vi "Liquid Crystal Display.vi"(0 "LINX Resource In":T1, 1 "string":string, 2 "Clear LCD?":u16, 3 "Data":u8[](array[numeric]), 4 "string 2":string, 5 "Error In":errorcluster) -> (14 "LINX Resource Out":T1, 15 "string":string, 17 "Response":u8[](array[numeric]), 18 "string 2":string, 19 "Error Out":errorcluster)   [LabVIEW 2020]
doc: "Creates a text to be displayed to LCD using the Arduino IDE."
uses:
  <vilib>/MakerHub/LINX/Private/Type Defs/LINX Ref.ctl
  <vilib>/MakerHub/LINX/Private/Type Defs/Platform.ctl
  <vilib>/MakerHub/LINX/Private/Type Defs/Interface.ctl
  <vilib>/MakerHub/LINX/Private/Device/Type Defs/LINX Device Config.ctl
  <vilib>/MakerHub/LINX/Private/Device/Type Defs/TCP Config.ctl
  <vilib>/MakerHub/LINX/Private/Device/Type Defs/Channels.ctl
  <vilib>/MakerHub/LINX/LMH-LINX.lvlib
  <vilib>/MakerHub/LINX/Private/Device/Device.lvlib
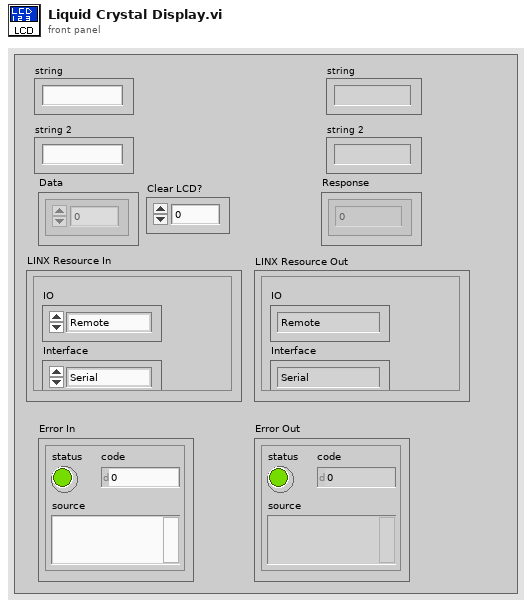
[diagram p1: front panel]
types:
  T1 = typedef "LMH-LINX.lvlib/LINX Ref.ctl" = cluster{"IO":T2, "Interface":T3, "LINX Device Config":T4}
  T2 = typedef "LMH-LINX.lvlib/Platform.ctl" = enum16{"Remote", "Local"}
  T3 = typedef "LMH-LINX.lvlib/Interface.ctl" = enum16{"Serial", "TCP"}
  T4 = typedef "LMH-LINX.lvlib/Device.lvlib/LINX Device Config.ctl" = cluster{"Interface":T3, "COM Port":refnum<visa-resource-name>, "TCP Configuration":T5, "Device Family":u8, "Device ID":u8, "Device Name":string, "TCP Ref":refnum<k5>, "Channels":T6}
  T5 = typedef "LMH-LINX.lvlib/Device.lvlib/TCP Config.ctl" = cluster{"IP Address":string, "Port":u16}
  T6 = typedef "LMH-LINX.lvlib/Channels.ctl" = cluster{"DI":u8[], "DO":u8[], "AI":u8[], "AO":u8[], "PWM":u8[], "QE":u8[], "UART":u8[], "I2C 2":u8[], "SPI":u8[], "CAN":u8[], "Servo":u8[], "AI Ref (V)":dbl, "AI Resolution (Bits)":u8, "AO Ref (V)":dbl, "AO Resolution (Bits)":u8}
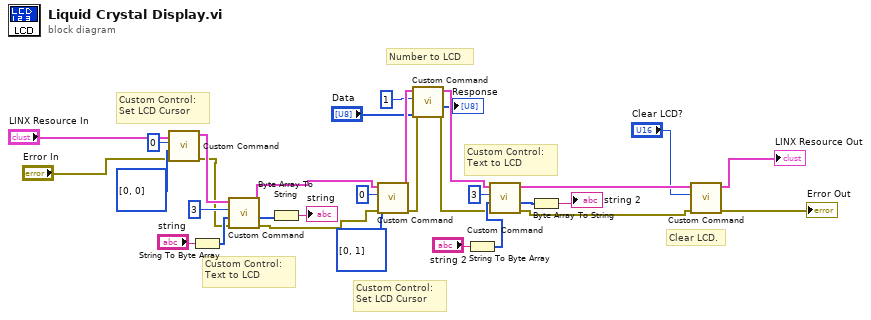
[diagram p0: block diagram]
diagram:
  # "Clear LCD."
  # "Number to LCD"
  # "Custom Control:\nText to LCD"
  # "Custom Control:\nSet LCD Cursor"
  # "Custom Control:\nText to LCD"
  # "Custom Control:\nSet LCD Cursor"
  n1 = call <vilib>:"Custom Command.vi"("Error In"="Error In", "Data"=u8[] [0, 0], "Custom Command Number"=u16 0, "LINX Resource"="LINX Resource In") -> ("Error Out"=w26:errorcluster, "LINX Resource"=w30:T1)  [unwired: 4 in, 2 out]
  n2 = String To Byte Array(string="string") -> (unsigned byte array=w27:u8[])
  n3 = call <vilib>:"Custom Command.vi"("Error In"=w26, "Data"=w27, "Custom Command Number"=u16 3, "LINX Resource"=w30) -> ("Error Out"=w16:errorcluster, "Response"=w25:u8[], "LINX Resource"=w15:T1)  [unwired: 4 in, 1 out]
  n4 = Byte Array To String(unsigned byte array=w25) -> (string=→"string":string)
  n5 = call <vilib>:"Custom Command.vi"("Error In"=w16, "Data"=u8[] [0, 1], "Custom Command Number"=u16 0, "LINX Resource"=w15) -> ("Error Out"=w9:errorcluster, "LINX Resource"=w12:T1)  [unwired: 4 in, 2 out]
  n6 = call <vilib>:"Custom Command.vi"("Error In"=w9, "Data"="Data", "Custom Command Number"=u16 1, "LINX Resource"=w12) -> ("Error Out"=w10:errorcluster, "Response"=→"Response":u8[], "LINX Resource"=w11:T1)  [unwired: 4 in, 1 out]
  n7 = String To Byte Array(string="string 2") -> (unsigned byte array=w20:u8[])
  n8 = call <vilib>:"Custom Command.vi"("Error In"=w10, "Data"=w20, "Custom Command Number"=u16 3, "LINX Resource"=w11) -> ("Error Out"=w4:errorcluster, "Response"=w17:u8[], "LINX Resource"=w5:T1)  [unwired: 4 in, 1 out]
  n9 = Byte Array To String(unsigned byte array=w17) -> (string=→"string 2":string)
  n10 = call <vilib>:"Custom Command.vi"("Error In"=w4, "Custom Command Number"="Clear LCD?", "LINX Resource"=w5) -> ("Error Out"=→"Error Out":errorcluster, "LINX Resource"=→"LINX Resource Out":T1)  [unwired: 5 in, 2 out]
